vi "Basic LED On Off.vi"() -> ()   [LabVIEW 2020]
panel:
  in  "stop":bool
  in  "Light Control":bool[](array[boolean])=[TRUE]
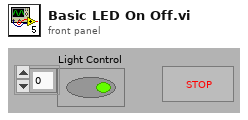
[diagram p1: front panel]
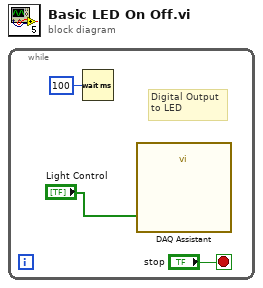
[diagram p0: block diagram]
diagram:
  n1 = while {
    stop <- "stop" stop-if-true
    # "Digital Output\nto LED"
    n2 = Wait (ms)(milliseconds to wait=u32 100) -> ()  [unwired: 1 out]
    n3 = call "DAQ Assistant"("data"="Light Control") -> ()  [unwired: 17 in, 2 out]
  }
